vi "Init blank volume table.vi"(8 "error in (no error)":errorcluster, 11 "Tomo in":refnum<class "Tomo.lvclass">) -> (0 "error out":errorcluster, 2 "blank volume table":dbl[][](array[numeric]), 3 "Tomo out":refnum<class "Tomo.lvclass">)   [LabVIEW 2012, in "Tomo.lvclass"]
uses:
  Tomo.lvclass
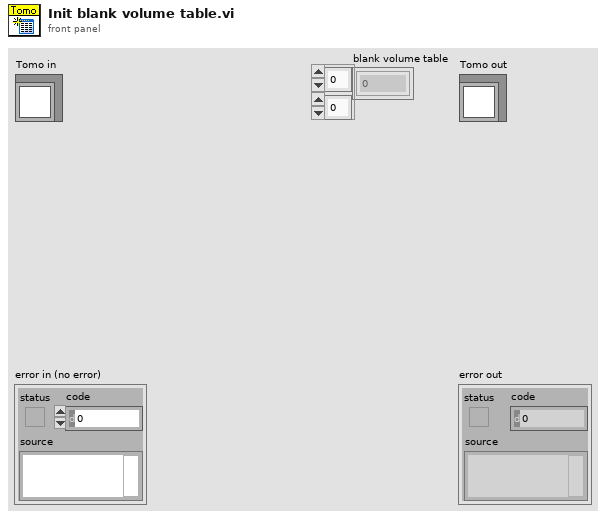
[diagram p1: front panel]
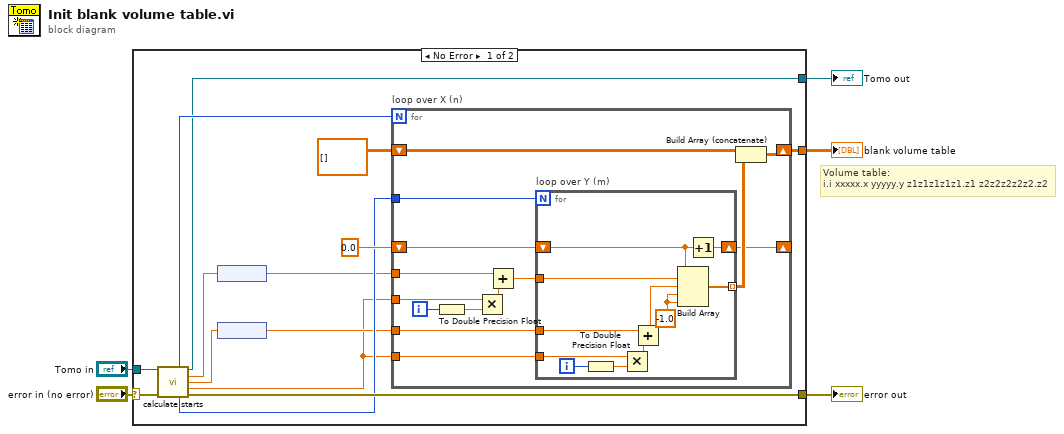
[diagram p0: block diagram]
diagram:
  # "Volume table: \ni.i xxxxx.x yyyyy.y z1z1z1z1z1.z1 z2z2z2z2z2.z2"
  n1 = case shown="No Error" "error in (no error)" {
    selector: "error in (no error)" -> [w16 w46]
    tunnel: [w15 w46] -> w4
    tunnel: [w6 w45] -> w2
    tunnel: "Tomo in" -> [w7 w45]
    tunnel: [w17 _] -> w1
    frame No Error {
      n2 = call-dynamic "calculate starts.vi"("Tomo in"=w7, "error in (no error)"=w16) -> ("x loop number"=w12:i32, "Tomo out"=w6:refnum<class "Tomo.lvclass">, "x_start"=w14:dbl[unit], "y_start"=w13:dbl[unit], "pretomo step size (px)"=w8:dbl, "y loop number"=w11:i32, "error out"=w15:errorcluster)  [unwired: 7 in]
      n3 = node(w14) -> (w10:dbl)
      n4 = node(w13) -> (w9:dbl)
      n5 = for "loop over X (n)" {
        N: w12 -> [_]
        tunnel: w11 -> [w33]
        shift-right: [w20] -> _
        shift-left: 0.0 -> [w31]
        tunnel: w10 -> [w27]
        tunnel: w8 -> [w26]
        tunnel: w9 -> [w25]
        tunnel: w8 -> [w24]
        shift-right: [w23] -> w17
        shift-left: dbl[][] [] -> [w21]
        i -> [w32]
        n6 = To Double Precision Float(number=w32) -> (double precision float=w29:dbl)
        n7 = Multiply(x=w26, y=w29) -> (x*y=w30:dbl)
        n8 = Add(x=w27, y=w30) -> (x+y=w28:dbl)
        n9 = for "loop over Y (m)" {
          N: w33 -> [_]
          shift-right: [w43] -> w20
          shift-left: w31 -> [w35]
          tunnel: w28 -> [w42]
          tunnel: w25 -> [w41]
          tunnel: w24 -> [w40]
          tunnel: [w36] -> w22 mode=indexing
          i -> [w44]
          w34 = -1.0
          n10 = To Double Precision Float(number=w44) -> (double precision float=w39:dbl)
          n11 = Multiply(x=w40, y=w39) -> (x*y=w38:dbl)
          n12 = Add(x=w41, y=w38) -> (x+y=w37:dbl)
          n13 = Build Array(w35, w42, w37, w34, w34) -> (w36:dbl[])
          n14 = Increment(x=w35) -> (x+1=w43:dbl)
        }
        n15 = Build Array (concatenate)(w21, w22) -> (w23:dbl[][])
      }
    }
    frame Error {
    }
  }
  "error out" <- w4
  "Tomo out" <- w2
  "blank volume table" <- w1
